vi "Test App Does Not Overwrite Configured Error Handler with Abstract Interface.vi"(8 "error in (no error)":errorcluster, 11 "Application Test in":refnum<class "Application Test.lvclass">) -> (0 "error out":errorcluster, 3 "Application Test out":refnum<class "Application Test.lvclass">)   [LabVIEW 2020, in "Application Test.lvclass"]
uses:
  Application Test.lvclass
  C:/Program Files (x86)/National Instruments/LabVIEW 2020/vi.lib/Asteme/LUnit/Test Case.lvclass
  Mock Process/Mock Process.lvclass
  C:/Users/anton/Documents/GitHub/Triarc-Framework/source/Framework/Process/Process.lvclass
  Mock Error Handler/Mock Error Handler.lvclass
  C:/Users/anton/Documents/GitHub/Triarc-Framework/source/Framework/Error Handler Interface/Error Handler Interface.lvclass
  Framework/Process/Process.lvclass/Process.ctl
  Framework/Application/Application.lvclass/Application.ctl
  <vilib>/Asteme/LUnit/Test Case.lvclass/Test Case.ctl
  <vilib>/Asteme/LUnit/LUnit Assertion Result.lvclass/LUnit Assertion Result.ctl
  Framework/Process/Public/Lifecycle/Get Lifecycle State.vi
  Framework/Process/Protected/Messaging/Enqueue Message.vi
  <vilib>/Utility/error.llb/Clear Errors.vi
  Framework/Process/Protected/SubVIs/Set Context.vi
  Framework/Application/Private/Add Process to Map.vi
  Framework/Process/Protected/Messaging/Request Message.vi
  Framework/Process/Private/SubVIs/Wait for finish.vi
  Framework/Process/Private/SubVIs/Set Lifecycle State.vi
  <vilib>/Asteme/LUnit/Palette/Pass.vi
  <vilib>/Asteme/LUnit/Palette/Fail.vi
  <vilib>/Asteme/LUnit/Variant to string.vi
  <vilib>/Asteme/LUnit/Set Assertion Type.vi
  <vilib>/AdvancedString/1D String Array to Delimited String.vi
  Framework/Process/Private/SubVIs/Enqueue Request Message.vi
  <vilib>/Asteme/LUnit/Add test result.vi
  <vilib>/Asteme/LUnit/LUnit Write Passed.vi
  <vilib>/Asteme/LUnit/LUnit Get Test Case.vi
  <vilib>/Asteme/LUnit/LUnit Write Message.vi
  <vilib>/Asteme/LUnit/LUnit Write Description.vi
  <vilib>/Asteme/LUnit/LUnit Write Assertion Type.vi
  <vilib>/Asteme/LUnit/Read Test Case Name.vi
  Framework/Application/Application.lvclass
  <vilib>/Utility/error.llb/Error Cluster From Error Code.vi
  Framework/Process/Private/SubVIs/Wait for Response Message.vi
  <vilib>/Asteme/LUnit/Assertion Result/LUnit Get Test Name.vi
  <vilib>/Utility/Data Type/Get Type Information.vi
  <vilib>/Utility/LVClass/Get LV Class Name.vi
  Framework/Process/Process.lvclass
  <vilib>/ErrorRing/Error Ring.xnode
  <vilib>/Asteme/LUnit/LUnit Assertion Result.lvclass
  <vilib>/Asteme/LUnit/Test Case.lvclass
  Support/Framework Test Support.lvlib
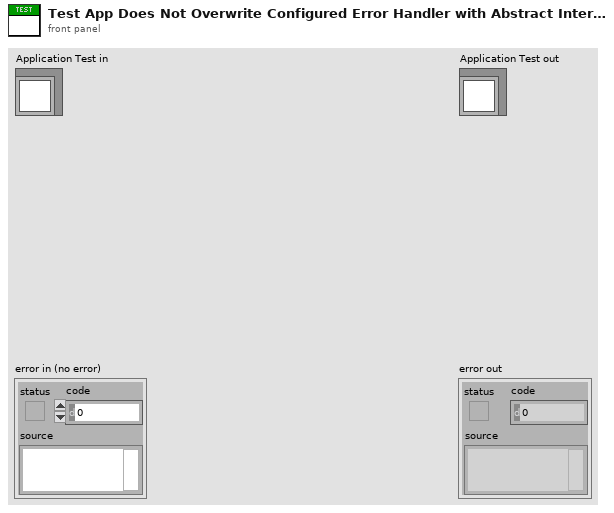
[diagram p1: front panel]
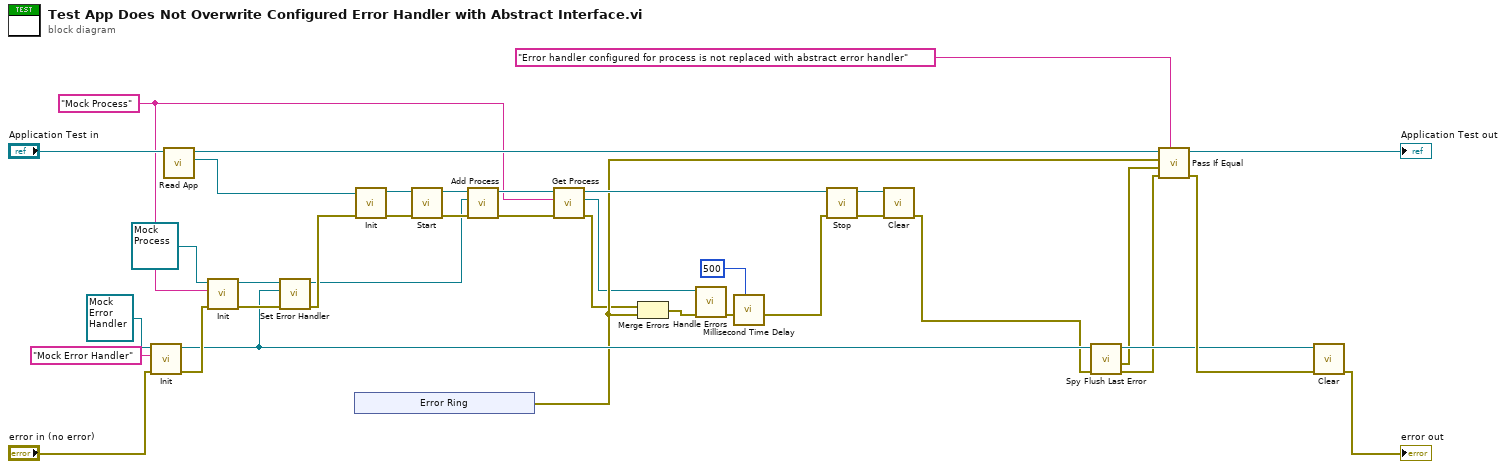
[diagram p0: block diagram]
diagram:
  w11 = "Mock Process" ("Name")
  n1 = call-dynamic "Init.vi"("error in (no error)"="error in (no error)", "Name"="Mock Error Handler", "Mock Error Handler In"=refnum<class "Mock Error Handler.lvclass"> refnum ("Mock Error Handler.lvclass")) -> ("error out"=w24:errorcluster, "Mock Error Handler Out"=w16:refnum<class "Mock Error Handler.lvclass">)  [unwired: 7 in]
  n2 = call "Read App.vi"("Application Test In"="Application Test in") -> ("App out"=w32:refnum<class "Application.lvclass">, "Application Test Out"=w37:refnum<class "Application Test.lvclass">)  [unwired: 8 in, 1 out]
  n3 = call-dynamic "Init.vi"("error in (no error)"=w24, "Name"=w11, "Mock Process In"=refnum<class "Mock Process.lvclass"> refnum ("Process In")) -> ("error out"=w36:errorcluster, "Mock Process Out"=w17:refnum<class "Mock Process.lvclass">)  [unwired: 7 in]
  n4 = call "Set Error Handler.vi"("error in (no error)"=w36, "Error Handler"=w16, "Process In"=w17) -> ("error out"=w25:errorcluster, "Process Out"=w5:refnum<class "Mock Process.lvclass">)  [unwired: 7 in]
  n5 = xnode "Error Ring"() -> ("error out"=w9:errorcluster)
  n6 = call-dynamic "Init.vi"("error in (no error)"=w25, "Process In"=w32) -> ("error out"=w19:errorcluster, "Process Out"=w31:refnum<class "Application.lvclass">)  [unwired: 8 in]
  n7 = call "Start.vi"("error in (no error)"=w19, "Process In"=w31) -> ("error out"=w18:errorcluster, "Process Out"=w20:refnum<class "Application.lvclass">)  [unwired: 8 in]
  n8 = call "Add Process.vi"("error in (no error)"=w18, "Process"=w5, "Rig In"=w20) -> ("error out"=w10:errorcluster, "Rig Out"=w30:refnum<class "Application.lvclass">)  [unwired: 7 in]
  n9 = call "Get Process.vi"("error in (no error)"=w10, "Process Name"=w11, "Rig In"=w30) -> ("error out"=w3:errorcluster, "App Process"=w4:refnum<class "Process.lvclass">, "Rig Out"=w12:refnum<class "Application.lvclass">)  [unwired: 6 in]
  n10 = Merge Errors(w3, w9) -> (w7:errorcluster)
  n11 = call-dynamic "Handle Errors.vi"("error in (no error)"=w7, "Process In"=w4) -> ("error out"=w8:errorcluster)  [unwired: 8 in, 1 out]
  n12 = call "Millisecond Time Delay.vi"("milliseconds to wait"=u32 500, "error in (no error)"=w8) -> ("error out"=w2:errorcluster)  [unwired: 7 in]
  n13 = call "Stop.vi"("error in (no error)"=w2, "Process In"=w12) -> ("error out"=w28:errorcluster, "Process Out"=w29:refnum<class "Application.lvclass">)  [unwired: 7 in, 1 out]
  n14 = call-dynamic "Clear.vi"("error in (no error)"=w28, "Application In"=w29) -> ("error out"=w1:errorcluster)  [unwired: 8 in, 1 out]
  n15 = call "Spy Flush Last Error.vi"("error in (no error)"=w1, "Mock Error Handler In"=w16) -> ("error out"=w14:errorcluster, "Error"=w13:errorcluster, "Mock Error Handler Out"=w15:refnum<class "Mock Error Handler.lvclass">)  [unwired: 7 in]
  n16 = call <vilib>:"Pass If Equal.vi"("Description"="Error handler configured for process is not replaced with abstract error handler", "error in (no error)"=w14, "Actual"=w13, "Expected"=w9, "Test Case In"=w37) -> ("error out"=w22:errorcluster, "Test Case Out"=→"Application Test out":refnum<class "Application Test.lvclass">)  [unwired: 5 in]
  n17 = call-dynamic "Clear.vi"("error in (no error)"=w22, "Mock Process In"=w15) -> ("error out"=→"error out":errorcluster)  [unwired: 8 in, 1 out]
